vi "Log.vi"(7 "Source":string, 8 "error in (no error)":errorcluster, 9 "Message":string, 10 "Level":T1, 11 "Process In":refnum<class "Process.lvclass">) -> (0 "error out":errorcluster, 3 "Process Out":refnum<class "Process.lvclass">)   [LabVIEW 2020, in "Process.lvclass"]
doc: "Enter a message into the system log by delegating the loging action to each of the set logging targets."
uses:
  Process.lvclass
  Logging/Protected/Level.ctl
  Logging/Logging.lvclass
  Process.lvclass/Process.ctl
  Public/Lifecycle/Get Lifecycle State.vi
  <vilib>/Utility/error.llb/Error Cluster From Error Code.vi
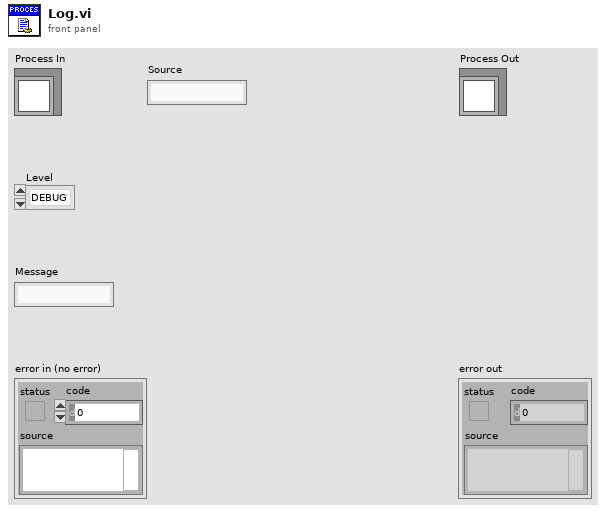
[diagram p1: front panel]
types:
  T1 = typedef "Logging.lvclass/Level.ctl" = enum16{"DEBUG", "INFO", "WARNING", "ERROR", "CRITICAL"}
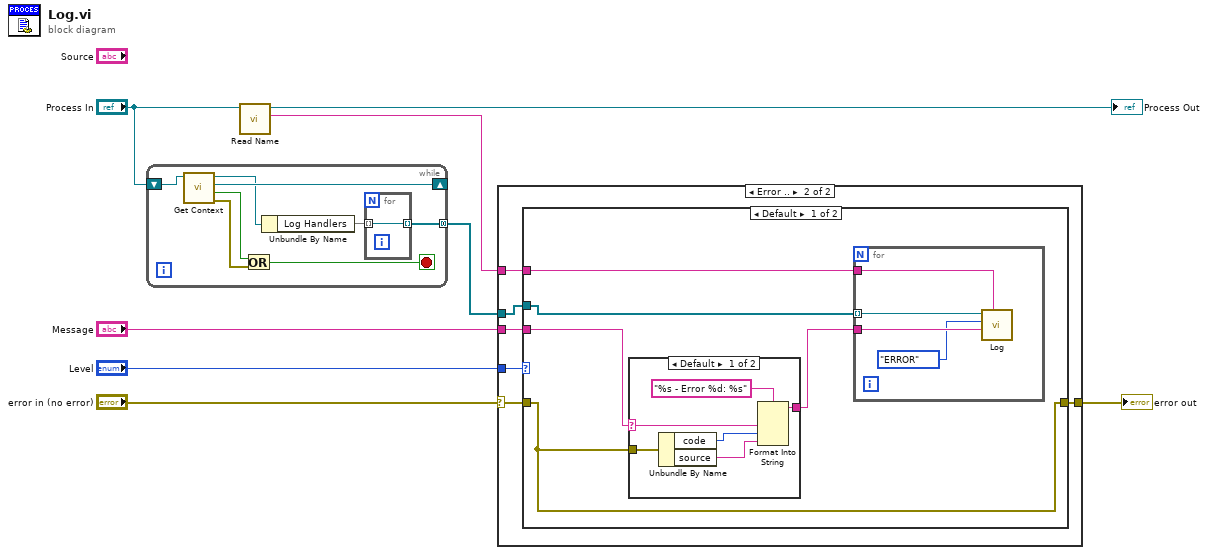
[diagram p0: block diagram]
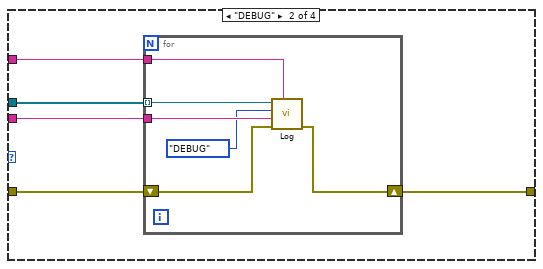
[diagram p3: hidden frame]
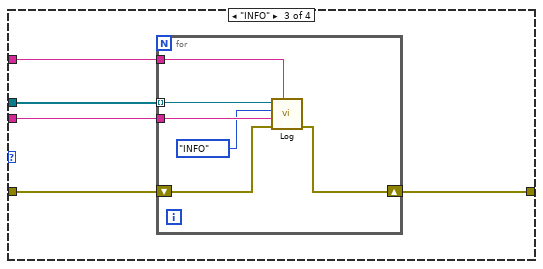
[diagram p4: hidden frame]
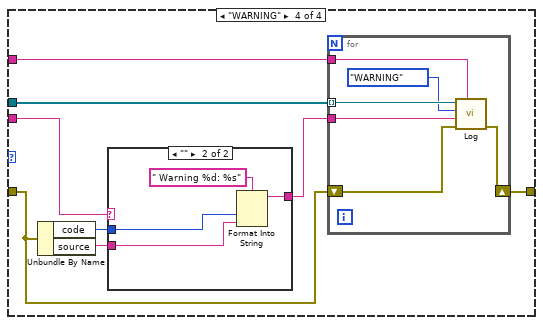
[diagram p5: hidden frame]
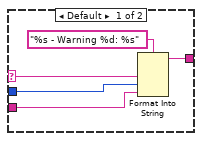
[diagram p6: hidden frame]
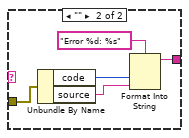
[diagram p7: hidden frame]
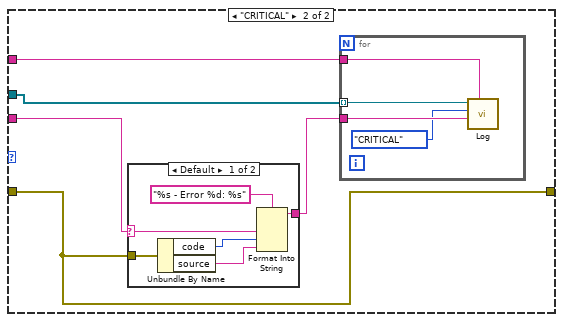
[diagram p8: hidden frame]
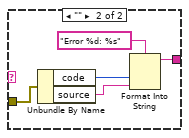
[diagram p9: hidden frame]
diagram:
  n1 = while {
    shift-right: [w12] -> _
    shift-left: "Process In" -> [w16]
    tunnel: [w10] -> w1 mode=concatenating
    stop <- w13 stop-if-true
    (unwired) set{refnum<class "Logging.lvclass">} {} ("Log Handlers")
    (unwired) set{refnum<class "Logging.lvclass">} {} ("Log Handlers")
    n2 = call "Get Context.vi"("Process In"=w16) -> ("error out"=w14:errorcluster, "Top Level?"=w15:bool, "Context"=w12:refnum<class "Process.lvclass">, "Process Out"=w9:refnum<class "Process.lvclass">)  [unwired: 7 in]
    n3 = Or(x=w15, y=w14) -> (x .or. y?=w13:bool)
    n4 = Unbundle By Name(w9) -> ("Log Handlers"=w11:set{refnum<class "Logging.lvclass">})
    n5 = for {
      tunnel: w11 -> [w17] mode=indexing
      tunnel: [w17] -> w10 mode=indexing
    }
  }
  n6 = call "Read Name.vi"("Process In"="Process In") -> ("Qualified Name"=w5:string, "Process Out"=→"Process Out":refnum<class "Process.lvclass">)  [unwired: 7 in, 2 out]
  n7 = case shown="Error .." "error in (no error)" {
    selector: "error in (no error)" -> [w19 w71]
    tunnel: w1 -> [w22 w74]
    tunnel: "Level" -> [w23 w75]
    tunnel: w5 -> [w21 w73]
    tunnel: "Message" -> [w20 w72]
    tunnel: [w18 w70] -> w6
    frame No Error {
      n8 = case shown="\"ERROR\", \"CRITICAL\"" w23 {
        tunnel: w22 -> [_ w25 w40 w52]
        tunnel: w21 -> [_ w29 w39 w54]
        tunnel: w20 -> [_ w28 w38 w47]
        tunnel: w19 -> [w24 w27 w37 w49]
        tunnel: [w24 w26 w36 w53] -> w18
        frame "ERROR", "CRITICAL" {
          # "Error and critical log messages are only recorded if there is an error"
        }
        frame "DEBUG" {
          n9 = for {
            tunnel: w25 -> [w35] mode=indexing
            tunnel: w29 -> [w34]
            tunnel: w28 -> [w33]
            shift-right: [w31] -> w26
            shift-left: w27 -> [w32]
            n10 = call-dynamic "Log.vi"("Source"=w34, "error in (no error)"=w32, "Message"=w33, "Level"=Level."DEBUG", "Logging In"=w35) -> ("error out"=w31:errorcluster)  [unwired: 5 in, 1 out]
          }
        }
        frame "INFO" {
          n11 = for {
            tunnel: w40 -> [w46] mode=indexing
            tunnel: w39 -> [w45]
            tunnel: w38 -> [w44]
            shift-right: [w42] -> w36
            shift-left: w37 -> [w43]
            n12 = call-dynamic "Log.vi"("Source"=w45, "error in (no error)"=w43, "Message"=w44, "Level"=Level."INFO", "Logging In"=w46) -> ("error out"=w42:errorcluster)  [unwired: 5 in, 1 out]
          }
        }
        frame "WARNING" {
          n13 = Unbundle By Name(w49) -> ("code"=w51:i32, "source"=w50:string)
          n14 = case shown="\"\"" w47 {
            selector: w47 -> [w55 _]
            tunnel: [w59 w63] -> w48
            tunnel: w51 -> [w57 w61]
            tunnel: w50 -> [w56 w60]
            frame Default {
              n15 = Format Into String(format string="%s - Warning %d: %s", w55, w57, w56) -> (resulting string=w59:string)  [unwired: 2 in, 1 out]
            }
            frame "" {
              n16 = Format Into String(format string=" Warning %d: %s", w61, w60) -> (resulting string=w63:string)  [unwired: 2 in, 1 out]
            }
          }
          n17 = for {
            tunnel: w52 -> [w69] mode=indexing
            tunnel: w54 -> [w68]
            tunnel: w48 -> [w67]
            shift-right: [w65] -> w53
            shift-left: w49 -> [w66]
            n18 = call-dynamic "Log.vi"("Source"=w68, "error in (no error)"=w66, "Message"=w67, "Level"=Level."WARNING", "Logging In"=w69) -> ("error out"=w65:errorcluster)  [unwired: 5 in, 1 out]
          }
        }
      }
    }
    frame Error {
      n19 = case shown="Default" w75 {
        tunnel: w74 -> [w80 w100]
        tunnel: w73 -> [w79 w99]
        tunnel: w72 -> [w77 w97]
        tunnel: w71 -> [w76 w96]
        tunnel: [w76 w96] -> w70
        frame Default {
          n20 = case shown="Default" w77 {
            selector: w77 -> [w81 _]
            tunnel: w76 -> [w86 w91]
            tunnel: [w82 w87] -> w78
            frame Default {
              n21 = Unbundle By Name(w86) -> ("code"=w84:i32, "source"=w83:string)
              n22 = Format Into String(format string="%s - Error %d: %s", w81, w84, w83) -> (resulting string=w82:string)  [unwired: 2 in, 1 out]
            }
            frame "" {
              n23 = Unbundle By Name(w91) -> ("code"=w89:i32, "source"=w88:string)
              n24 = Format Into String(format string="Error %d: %s", w89, w88) -> (resulting string=w87:string)  [unwired: 2 in, 1 out]
            }
          }
          n25 = for {
            tunnel: w80 -> [w95] mode=indexing
            tunnel: w79 -> [w94]
            tunnel: w78 -> [w93]
            n26 = call-dynamic "Log.vi"("Source"=w94, "Message"=w93, "Level"=Level."ERROR", "Logging In"=w95) -> ()  [unwired: 6 in, 2 out]
          }
        }
        frame "CRITICAL" {
          n27 = case shown="Default" w97 {
            selector: w97 -> [w101 _]
            tunnel: w96 -> [w106 w111]
            tunnel: [w102 w107] -> w98
            frame Default {
              n28 = Unbundle By Name(w106) -> ("code"=w104:i32, "source"=w103:string)
              n29 = Format Into String(format string="%s - Error %d: %s", w101, w104, w103) -> (resulting string=w102:string)  [unwired: 2 in, 1 out]
            }
            frame "" {
              n30 = Unbundle By Name(w111) -> ("code"=w109:i32, "source"=w108:string)
              n31 = Format Into String(format string="Error %d: %s", w109, w108) -> (resulting string=w107:string)  [unwired: 2 in, 1 out]
            }
          }
          n32 = for {
            tunnel: w100 -> [w115] mode=indexing
            tunnel: w99 -> [w114]
            tunnel: w98 -> [w113]
            n33 = call-dynamic "Log.vi"("Source"=w114, "Message"=w113, "Level"=Level."CRITICAL", "Logging In"=w115) -> ()  [unwired: 6 in, 2 out]
          }
        }
      }
    }
  }
  "error out" <- w6
